vi "toInstrumentScript.vi"(8 "error in (no error)":errorcluster, 11 "device in":refnum<class "device.lvclass">) -> (0 "error out":errorcluster, 2 "instrument_ScriptXml":refnum<class "xmlNode.lvclass">, 3 "device out":refnum<class "device.lvclass">)   [LabVIEW 2011, in "Tools.lvlib" / "DatabaseHelpers.lvlib" / "device.lvclass"]
uses:
  device.lvclass
  xmlNode/xmlNode.lvclass
  device.lvclass/device.ctl
  Scripting/ScriptingEvent/ScriptEventList/ScriptEventList.lvclass
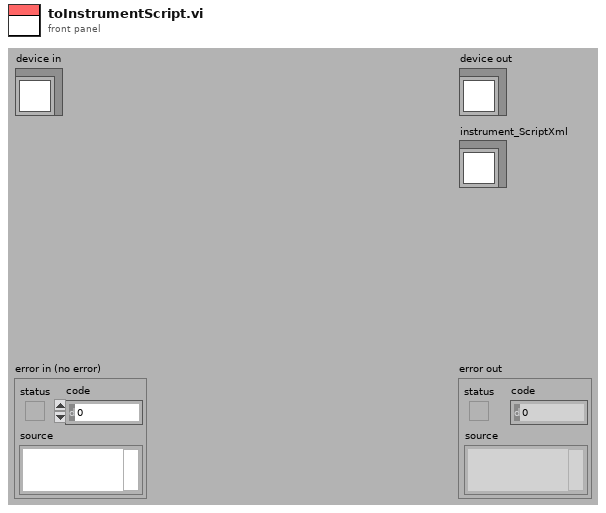
[diagram p1: front panel]
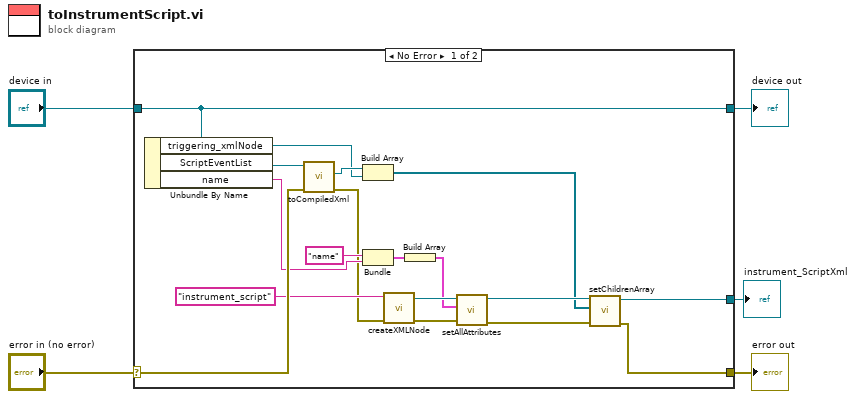
[diagram p0: block diagram]
diagram:
  n1 = case shown="No Error" "error in (no error)" {
    selector: "error in (no error)" -> [w21 w25]
    tunnel: [w8 w25] -> w4
    tunnel: [w23 w24] -> w2
    tunnel: "device in" -> [w23 w24]
    tunnel: [w7 _] -> w1
    frame No Error {
      n2 = Unbundle By Name(w23) -> ("triggering_xmlNode"=w10:refnum<class "xmlNode.lvclass">, "ScriptEventList"=w22:refnum<class "ScriptEventList.lvclass">, "name"=w16:string)
      n3 = call "toCompiledXml.vi"("error in (no error)"=w21, "ScriptEventList in"=w22) -> ("error out"=w6:errorcluster, "compiledXml"=w11:refnum<class "xmlNode.lvclass">)  [unwired: 7 in, 1 out]
      n4 = Build Array(w11, w10) -> (w9:refnum<class "xmlNode.lvclass">[])
      n5 = Bundle("name", "name"=w16) -> (w15:cluster{string, "name":string})  [unwired: 1 in]
      n6 = call "createXMLNode.vi"("error in (no error)"=w6, "name"="instrument_script") -> ("error out"=w18:errorcluster, "xmlNode out"=w19:refnum<class "xmlNode.lvclass">)  [unwired: 8 in]
      n7 = Build Array(w15) -> (w14:cluster{string, "name":string}[])
      n8 = call-dynamic "setAllAttributes.vi"("error in (no error)"=w18, "attributes"=w14, "xmlNode in"=w19) -> ("error out"=w12:errorcluster, "xmlNode out"=w13:refnum<class "xmlNode.lvclass">)  [unwired: 7 in]
      n9 = call-dynamic "setChildrenArray.vi"("error in (no error)"=w12, "Children"=w9, "xmlNode.lvclass in"=w13) -> ("error out"=w8:errorcluster, "xmlNode.lvclass out"=w7:refnum<class "xmlNode.lvclass">)  [unwired: 7 in]
    }
    frame Error {
    }
  }
  "error out" <- w4
  "device out" <- w2
  "instrument_ScriptXml" <- w1
